vi "Finalize To Settings.vi"(8 "error in (no error)":errorcluster, 11 "Core Transfer Configuration in":refnum<class "Core Transfer Configuration.lvclass">) -> (0 "error out":errorcluster, 1 "settings version":T1, 2 "settings":cluster{"key":string, "value":string}[](array[cluster]), 3 "Core Transfer Configuration out":refnum<class "Core Transfer Configuration.lvclass">)   [LabVIEW 2017, in "DSF Core.lvlib" / "Core Transfer Configuration.lvclass"]
uses:
  Core Transfer Configuration.lvclass
  Typedefs/DSF Version Info.ctl
  Core Transfer Configuration.lvclass/Core Transfer Configuration.ctl
  DSF Core.lvlib
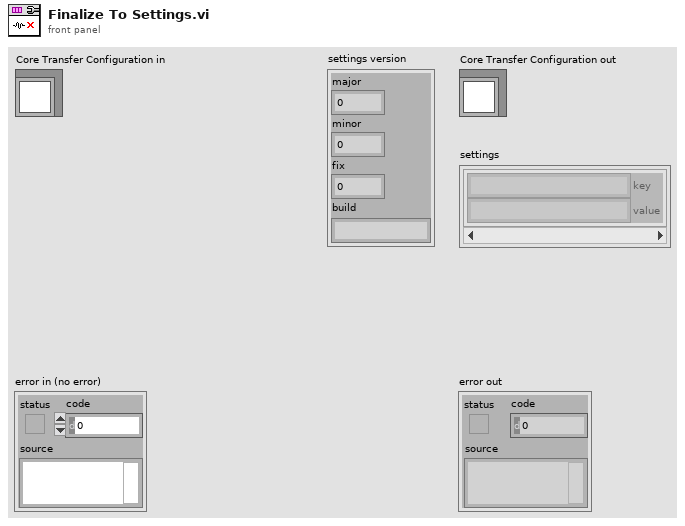
[diagram p1: front panel]
types:
  T1 = typedef "DSF Core.lvlib/DSF Version Info.ctl" = cluster{"major":u32, "minor":u32, "fix":u32, "build":string}
  T2 = typedef "DSF Core.lvlib/DSF Core Transfer Configuration.ctl" = cluster{"name":string}
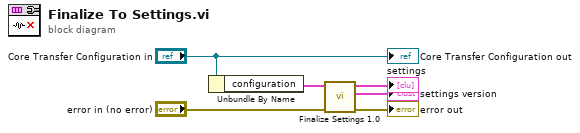
[diagram p0: block diagram]
diagram:
  n1 = Unbundle By Name("Core Transfer Configuration in") -> ("configuration"=w2:T2)
  n2 = call "Finalize Settings 1.0.vi"("error in (no error)"="error in (no error)", "configuration 1.0"=w2) -> ("error out"=→"error out":errorcluster, "settings version"=→"settings version":T1, "settings 1.0"=→"settings":cluster{"key":string, "value":string}[])  [unwired: 7 in]
  "Core Transfer Configuration out" <- "Core Transfer Configuration in"
